vi "Test header flatten.vi"() -> ()   [LabVIEW 2021]
uses:
  typedef/FIFO Header.ctl
  CIFCore/Common/Utilities/Add Error.vi
  <vilib>/CIF Foundation/CIF Utilities/Errors/Append Error Location.vi
  ChannelCommon.lvlib
panel:
  in  "error in":errorcluster
  out "Flatten Header out":u8[](array[numeric])
  out "error out":errorcluster
  out "Header out":T1
  in  "Header in":T1={"Length"=123, "T0"=1423, "T_Out"=5245, "T_Tx"=5, "Ctr"=875, "ClockID"=0}
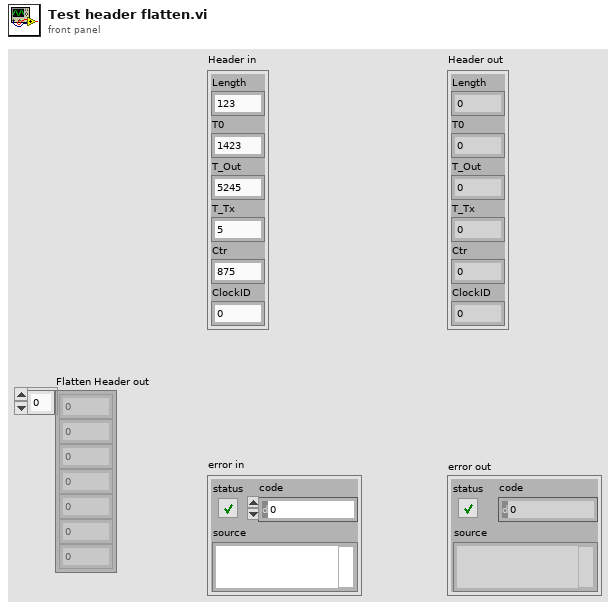
[diagram p1: front panel]
types:
  T1 = typedef "ChannelCommon.lvlib/FIFO Header.ctl" = cluster{"Length":u64, "T0":i64, "T_Out":i64, "T_Tx":i64, "Ctr":u64, "ClockID":u8}
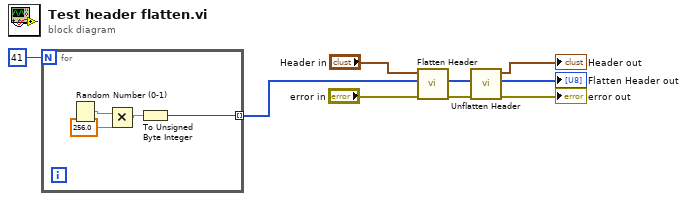
[diagram p0: block diagram]
diagram:
  n1 = for {
    N: 41 ("Numeric") -> [_]
    tunnel: [w10] -> w3 mode=indexing
    n2 = Random Number (0-1)() -> (number: 0 to 1=w13:dbl)
    n3 = Multiply(x=w13, y=256.0) -> (x*y=w11:dbl)
    n4 = To Unsigned Byte Integer(number=w11) -> (unsigned 8bit integer=w10:u8)
  }
  n5 = call "Flatten Header.vi"("error in"="error in", "Flattened Data in"=w3, "Header in"="Header in") -> ("error out"=w8:errorcluster, "Flattened Data out"=w9:u8[])  [unwired: 6 in, 1 out]
  n6 = call "Unflatten Header.vi"("error in"=w8, "Flattened Data in"=w9) -> ("error out"=→"error out":errorcluster, "Flatten Data out"=→"Flatten Header out":u8[], "Header out"=→"Header out":T1)  [unwired: 7 in]
